vi "Convert C to F.vi"(1 "deg C":dbl) -> (0 "deg F":dbl)   [LabVIEW 2015]
doc: "This VI converts a Celsius reading to a Fahrenheit reading."
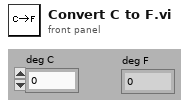
[diagram p1: front panel]
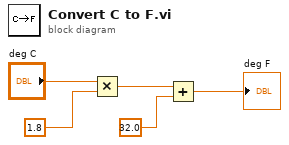
[diagram p0: block diagram]
diagram:
  n1 = Multiply(x="deg C", y=1.8) -> (x*y=w3:dbl)
  n2 = Add(x=w3, y=32.0) -> (x+y=→"deg F":dbl)
